vi "Error.vi"(8 "error in (no error)":errorcluster, 10 "ErrorCode":u32, 11 "ReturnValue":u32) -> (0 "Error_Out":T1, 2 "Error?":bool)   [LabVIEW 2015]
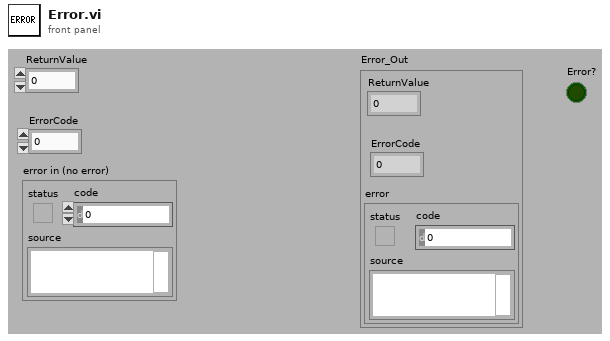
[diagram p1: front panel]
types:
  T1 = cluster{"ReturnValue":u32, "ErrorCode":u32, "error ":errorcluster}
  T2 = cluster{"ReturnValue":u32, "ErrorCode":u32, "error in (no error)":errorcluster}
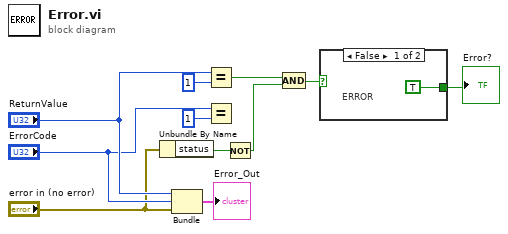
[diagram p0: block diagram]
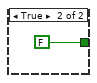
[diagram p2: hidden frame]
diagram:
  n1 = Unbundle By Name("error in (no error)") -> ("status"=w4:bool)
  n2 = Bundle("ReturnValue"="ReturnValue", "ErrorCode"="ErrorCode", "error in (no error)"="error in (no error)") -> (→"Error_Out":T2)  [unwired: 1 out]
  n3 = Equal?(x="ReturnValue", y=u32 1) -> (x = y?=w6:bool)
  n4 = Equal?(x="ErrorCode", y=u32 1) -> ()  [unwired: 1 out]
  n5 = Not(x=w4) -> (.not. x?=w3:bool)
  n6 = Compound Arithmetic op=AND(w6, w3) -> (w2:bool)
  n7 = case shown="False" w2 {
    tunnel: [TRUE FALSE] -> w1
    frame False {
      # "ERROR"
    }
    frame True {
    }
  }
  "Error?" <- w1
